vi "Begin.vi"(11 "Image Size":T1=enum."160x120") -> (0 "error out":errorcluster)   [LabVIEW 2012]
doc: "Called before other user functions, this VI is expected to open initial I/O refnums, load in file data, and do all program initialization. Notice that the <B>error out</B> terminal is simply used for data flow. Wiring it to other structures or subVIs ensures that this VI runs first."
uses:
  <vilib>/Rock Robotics/WPI/Camera/WPI_CameraImageSize.ctl
  <vilib>/Rock Robotics/SystemInterfaces/DIO/FPGA_DIOPWMChannel.ctl
  <vilib>/Rock Robotics/WPI/Camera/WPI_CameraWhite Balance Values.ctl
  <vilib>/Rock Robotics/WPI/Camera/WPI_CameraExposure Values.ctl
  <vilib>/Rock Robotics/WPI/Camera/WPI_CameraFrameRate.ctl
  <vilib>/Rock Robotics/WPI/DriverStation/WPI_DriverStationRobotMode2.ctl
  <vilib>/Rock Robotics/WPI/Joystick/WPI_JoystickDeviceEnum.ctl
  <vilib>/Rock Robotics/SystemInterfaces/Typedef/FPGA_TypedefSolenoidModule.ctl
  <vilib>/Rock Robotics/WPI/Solenoid/WPI_SolenoidChannel.ctl
  <vilib>/Rock Robotics/WPI/Encoder/WPI_EncoderType.ctl
  <vilib>/Rock Robotics/SystemInterfaces/DIO/FPGA_DIOChannel.ctl
  <vilib>/Rock Robotics/SystemInterfaces/Typedef/FPGA_TypedefDigitalModule.ctl
  <vilib>/Rock Robotics/WPI/SafetyOutput/WPI_SafetyOutputConfigMenu.ctl
  <vilib>/Rock Robotics/WPI/RobotDrive/WPI_RobotDriveOpen2MotorWithJaguar.vi
  F:/Team 1699 2013 robot code/Team 1699 2013 Robot Project V1a/Robot Global Data.vi
  <vilib>/Rock Robotics/WPI/Solenoid/WPI_SolenoidOpenSingle.vi
  <vilib>/Rock Robotics/WPI/Counter/WPI_CounterDigitalInputToDigitalSource.vi
  <vilib>/Rock Robotics/WPI/MotorControl/WPI_MotorControlOpen Talon.vi
  <vilib>/Utility/config.llb/Read Key (Double).vi
  <vilib>/Rock Robotics/SystemInterfaces/DIO/FPGA_DIORelayChannel.ctl
  <vilib>/Utility/config.llb/NI_LVConfig.lvlib
panel:
  out "found?":bool
  out "1699-preferences.ini":string[][](array[string])
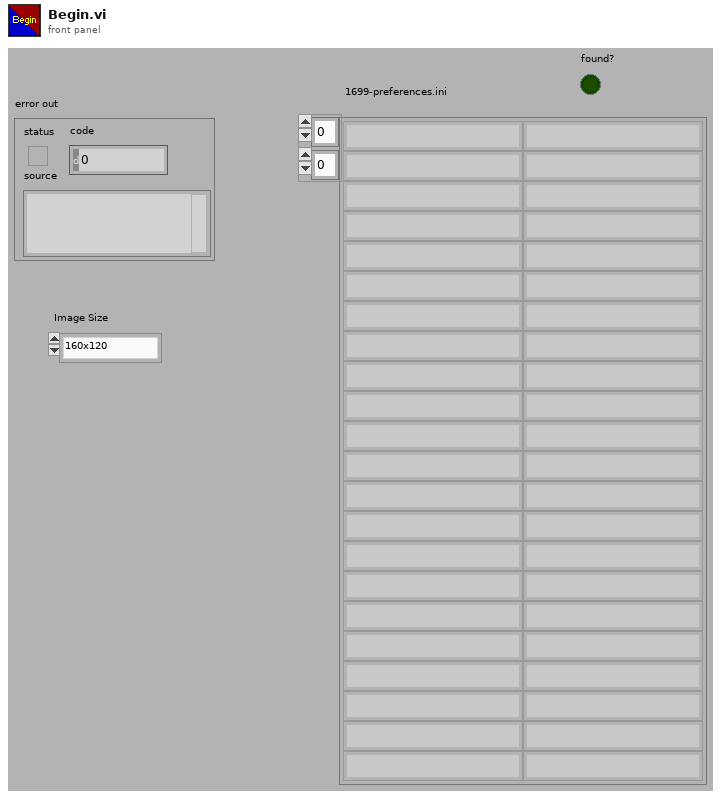
[diagram p1: front panel]
types:
  T1 = typedef "WPI_CameraImageSize.ctl" = enum16{"640x480", "320x240", "160x120"}
  T2 = typedef "WPI_SafetyOutputConfigMenu.ctl" = enum16{"Enable", "Disable"}
  T3 = typedef "FPGA_TypedefDigitalModule.ctl" = enum16{"Digital Module 1", "Digital Module 2"}
  T4 = typedef "FPGA_DIOPWMChannel.ctl" = enum8{"PWM 1", "PWM 2", "PWM 3", "PWM 4", "PWM 5", "PWM 6", "PWM 7", "PWM 8", "PWM 9", "PWM 10", "Invalid"}
  T5 = typedef "FPGA_DIOChannel.ctl" = enum8{"DIO 1", "DIO 2", "DIO 3", "DIO 4", "DIO 5", "DIO 6", "DIO 7", "DIO 8", "DIO 9", "DIO 10", "DIO 11", "DIO 12", "DIO 13", "DIO 14", "Invalid"}
  T6 = typedef "WPI_EncoderType.ctl" = enum16{"1x", "2x", "4x"}
  T7 = typedef "WPI_SolenoidChannel.ctl" = enum8{"Solenoid 1", "Solenoid 2", "Solenoid 3", "Solenoid 4", "Solenoid 5", "Solenoid 6", "Solenoid 7", "Solenoid 8", "Invalid"}
  T8 = typedef "FPGA_TypedefSolenoidModule.ctl" = enum16{"Solenoid Module 1", "Solenoid Module 2"}
  T9 = typedef "WPI_JoystickDeviceEnum.ctl" = enum16{"USB 1", "USB 2", "USB 3", "USB 4", "Kinect 1", "Kinect 2"}
  T10 = typedef "WPI_DriverStationRobotMode2.ctl" = enum16{"Autonomous Disabled", "Autonomous Enabled", "Teleop Disabled", "Teleop Enabled", "Timeout", "Finish", "Test Disabled", "Test Enabled"}
  T11 = typedef "WPI_CameraFrameRate.ctl" = u32
  T12 = typedef "WPI_CameraExposure Values.ctl" = enum16{"Auto", "Flicker-free 50 Hz", "Flicker-free 60 Hz", "Hold current"}
  T13 = typedef "WPI_CameraWhite Balance Values.ctl" = enum16{"Auto", "Fixed indoor", "Fixed outdoor 1", "Fixed outdoor 2", "Fixed fluorescent 1", "Fixed fluorescent 2", "Hold current"}
  T14 = typedef "WPI_DigitalInputDevRef.ctl" = cluster{"DevStatus":errorcluster, "DIO Channel":T5, "Digital Module":T3}
  T15 = typedef "FPGA_CounterEncoderSourceConvertionLVSourceType.ctl" = cluster{"DevStatus":errorcluster, "AnalogTriggerMode?":bool, "DigitalMode":cluster{"Digital Module":T3, "DIO Channel":T16}, "AnalogTriggerMode":cluster{"AnalogTriggerIndex":T17, "OutputType":T18}}
  T16 = typedef "FPGA_DIODigitalSourceChannel.ctl" = enum8{"DIO 1", "DIO 2", "DIO 3", "DIO 4", "DIO 5", "DIO 6", "DIO 7", "DIO 8", "DIO 9", "DIO 10", "DIO 11", "DIO 12", "DIO 13", "DIO 14", "Disabled"}
  T17 = typedef "FPGA_AnalogTriggerIndex.ctl" = enum8{"Trig 0", "Trig 1", "Trig 2", "Trig 3", "Trig 4", "Trig 5", "Trig 6", "Trig 7", "Invalid"}
  T18 = typedef "FPGA_AnalogTriggerOutType.ctl" = enum16{"InWindow", "TriggerState", "Rising", "Falling"}
  T19 = typedef "WPI_EncoderDevRef.ctl" = cluster{"DevStatus":errorcluster, "EncoderIndex":T20, "CounterIndex":T21, "DistancePerCount":dbl, "Decoding Type":T6}
  T20 = typedef "FPGA_EncoderIdx.ctl" = enum8{"Enc 0", "Enc 1", "Enc 2", "Enc 3", "Invalid"}
  T21 = typedef "FPGA_CounterCtrSystemIndex.ctl" = enum8{"Ctr 0", "Ctr 1", "Ctr 2", "Ctr 3", "Ctr 4", "Ctr 5", "Ctr 6", "Ctr 7", "Invalid"}
  T22 = cluster{"[0]":dbl, "[1]":dbl, "[2]":dbl, "[3]":dbl, "[4]":dbl, "[5]":dbl, "[6]":dbl, "[7]":dbl, "[8]":dbl, "[9]":dbl, "[10]":dbl, "[11]":dbl, "[12]":dbl, "[13]":dbl, "[14]":dbl, "[15]":dbl, "[16]":dbl, "[17]":dbl, "[18]":dbl, "[19]":dbl}
  T23 = typedef "FPGA_DIORelayChannel.ctl" = enum8{"Relay 1", "Relay 2", "Relay 3", "Relay 4", "Relay 5", "Relay 6", "Relay 7", "Relay 8", "Invalid"}
  T24 = typedef "WPI_CompressorDevRef.ctl" = cluster{"DevStatus":errorcluster, "DigitalInputDevRef":T14, "RelayDevRef":T25}
  T25 = typedef "WPI_RelayDevRef.ctl" = cluster{"DevStatus":errorcluster, "Relay Channel":T23, "Digital Module":T3, "Relay Direction":T26}
  T26 = typedef "WPI_RelayDirection.ctl" = enum16{"Both directions", "Forward only", "Reverse only"}
  T27 = typedef "WPI_MotorControlDeviceRef.ctl" = cluster{"DeviceStatus":errorcluster, "Type":enum16{"PWM", "CAN"}, "PWM":cluster{"Digital Module":T3, "PWM Channel":T4, "DeadBand":T28}, "CAN":cluster{"Device Number":u8, "Control Mode":T29, "Semaphore":T30, "Max Vout":dbl}, "Invert":bool, "TransformRef":T31, "InvTransformRef":T31}
  T28 = typedef "WPI_PWMDeadband.ctl" = cluster{"Name":string, "maxPositivePwm":i32, "minPositivePwm":i32, "centerPwm":i32, "maxNegativePwm":i32, "minNegativePwm":i32, "angularRange":u16}
  T29 = typedef "WPI_CANJaguar_ControlMode.ctl" = enum8{"Percent VBus", "Current", "Speed", "Position", "Voltage"}
  T30 = typedef "Semaphore RefNum" = refnum<k1>
  T31 = typedef "WPI_PWMTransform_ConPane.ctl" = refnum<vi>
  T32 = typedef "NI_LVConfig.lvlib/Config Data RefNum.ctl" = refnum<k1>
  T33 = typedef "WPI_JoystickDevRef.ctl" = cluster{"Device":T9}
  T34 = typedef "WPI_CameraDevRef.ctl" = cluster{"Camera Address":string, "CameraStatus":errorcluster, "Acquire Image Notifier":refnum<notifier>}
  T35 = typedef "WPI_RobotDriveDevRef.ctl" = cluster{"DevStatus":errorcluster, "Motors[]":T27[], "Square Inputs":bool, "Max Output":dbl, "Isochronous":bool}
  T36 = typedef "WPI_SolenoidDevRef.ctl" = cluster{"DevStatus":errorcluster, "Solenoid Module":T8, "Forward Solenoid Channel":T7, "Reverse Solenoid Channel":T7}
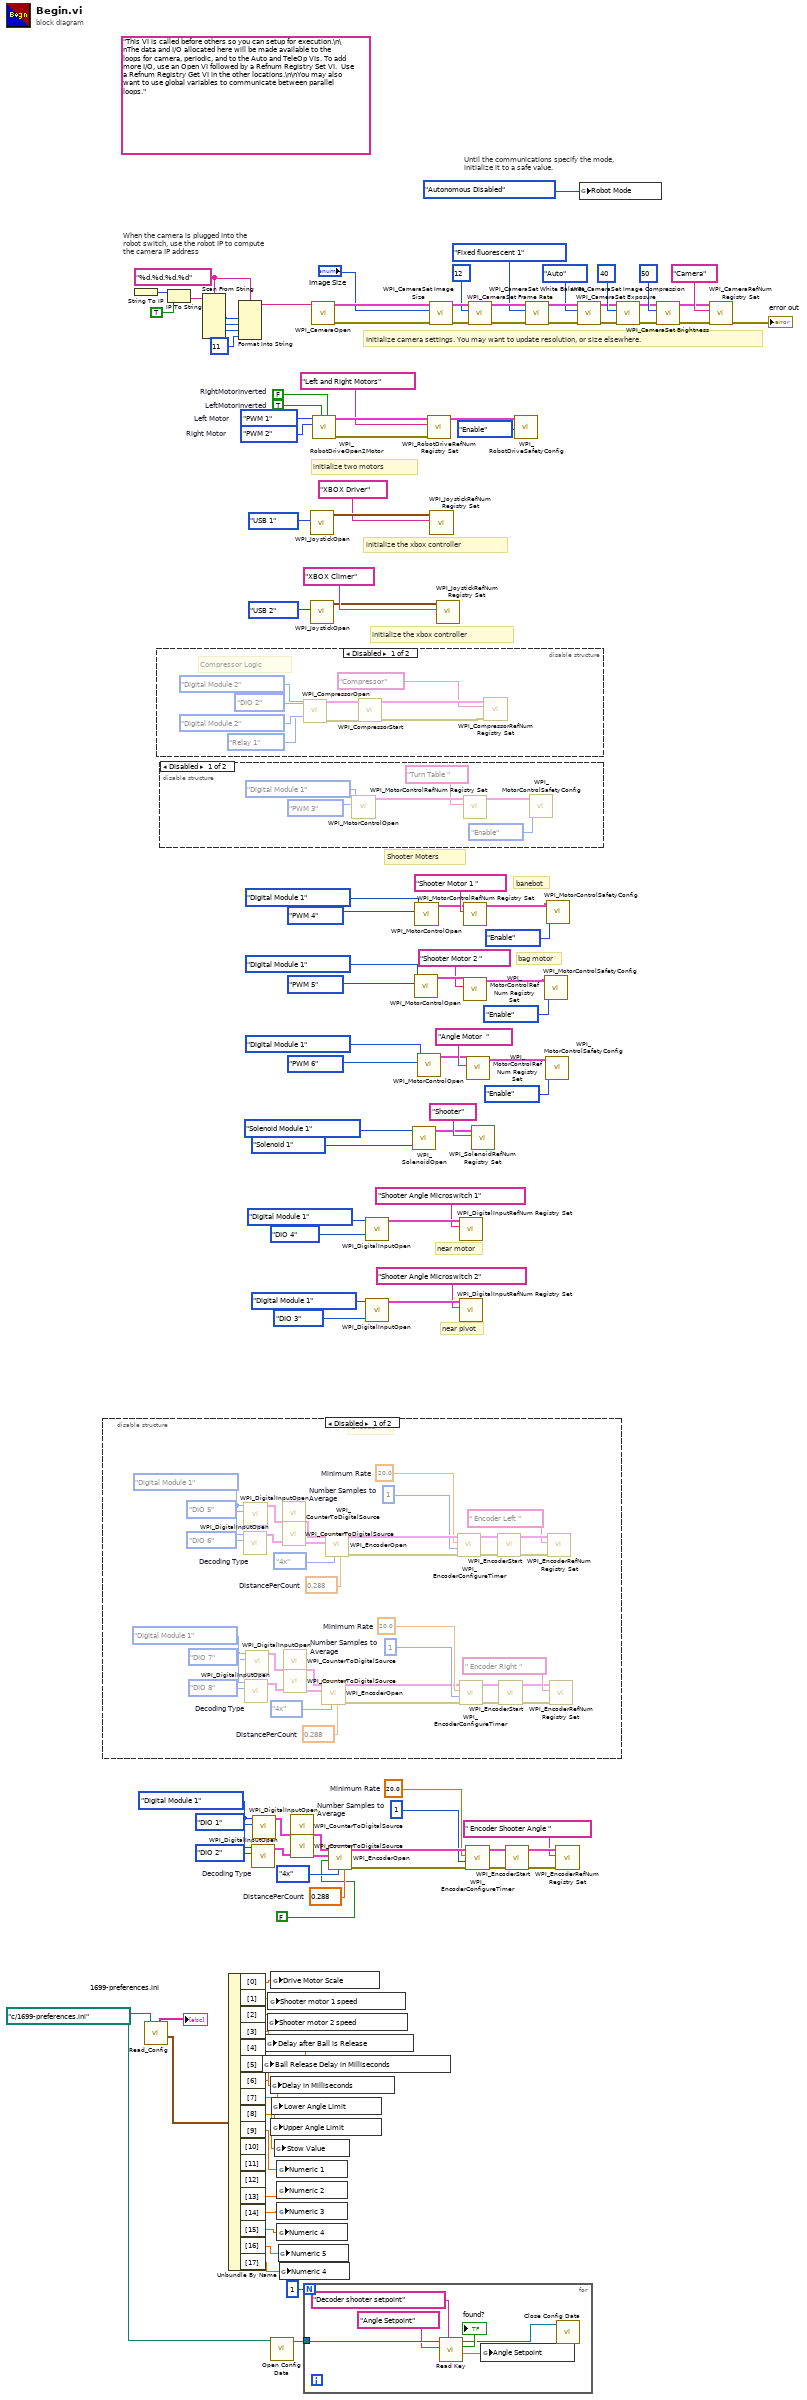
[diagram p0: block diagram]
diagram:
  w10 = path "c:/1699-preferences.ini" ("configuration file path")
  w48 = FPGA_TypedefDigitalModule."Digital Module 1" ("Digital Module (Module 1)")
  w55 = 0.288  # DistancePerCount
  w56 = WPI_EncoderType."4x"  # Decoding Type
  w57 = u8 1  # Number Samples to Average
  w58 = 20.0  # Minimum Rate
  w81 = "%d.%d.%d.%d" ("format string")
  (unwired) "This VI is called before others so you can setup for execution.\n\nThe data and I/O allocated here will be made available to the loops for camera, periodic, and to the Auto and TeleOp VIs. To add more I/O, use an Open VI followed by a Refnum Registry Set VI.  Use a Refnum Registry Get VI in the other locations.\n\nYou may also want to use global variables to communicate between parallel loops."
  w92 = FPGA_DIOPWMChannel."PWM 2"  # Right Motor
  w93 = FPGA_DIOPWMChannel."PWM 1"  # Left Motor
  w115 = TRUE  # LeftMotorInverted
  w116 = FALSE  # RightMotorInverted
  # "banebot"
  # "bag motor"
  # "Shooter Moters"
  # "initialize the xbox controller"
  # "near motor"
  # "near pivot"
  # "initialize the xbox controller"
  # "Until the communications specify the mode,\ninitialize it to a safe value."
  # "When the camera is plugged into the\nrobot switch, use the robot IP to compute\nthe camera IP address"
  # "initialize two motors"
  # "Initialize camera settings. You may want to update resolution, or size elsewhere."
  n1 = disable-structure shown="Disabled" {
    frame Disabled {
      w134 = FPGA_TypedefDigitalModule."Digital Module 1" ("Digital Module (Module 1)")
      w127 = 0.288  # DistancePerCount
      w126 = WPI_EncoderType."4x"  # Decoding Type
      w125 = u8 1  # Number Samples to Average
      w124 = 20.0  # Minimum Rate
      w135 = FPGA_TypedefDigitalModule."Digital Module 1" ("Digital Module (Module 1)")
      w142 = 0.288  # DistancePerCount
      w143 = WPI_EncoderType."4x"  # Decoding Type
      w144 = u8 1  # Number Samples to Average
      w145 = 20.0  # Minimum Rate
      # "Encoder"
      n2 = call <vilib>:"WPI_DigitalInputOpen.vi"("DIO Channel"=FPGA_DIOChannel."DIO 6", "Digital Module (Module 1)"=w135) -> ("DigitalInputDevRef"=w139:T14)  [unwired: 8 in, 1 out]
      n3 = call <vilib>:"WPI_DigitalInputOpen.vi"("DIO Channel"=FPGA_DIOChannel."DIO 5", "Digital Module (Module 1)"=w135) -> ("DigitalInputDevRef"=w138:T14)  [unwired: 8 in, 1 out]
      n4 = call <vilib>:"WPI_DigitalInputOpen.vi"("DIO Channel"=FPGA_DIOChannel."DIO 8", "Digital Module (Module 1)"=w134) -> ("DigitalInputDevRef"=w130:T14)  [unwired: 8 in, 1 out]
      n5 = call <vilib>:"WPI_DigitalInputOpen.vi"("DIO Channel"=FPGA_DIOChannel."DIO 7", "Digital Module (Module 1)"=w134) -> ("DigitalInputDevRef"=w131:T14)  [unwired: 8 in, 1 out]
      n6 = call-poly <vilib>:"WPI_CounterToDigitalSource.vi"("DigitalInputDevRef"=w138) -> ("Digital Source"=w140:T15)  [unwired: 6 in]
      n7 = call-poly <vilib>:"WPI_CounterToDigitalSource.vi"("DigitalInputDevRef"=w139) -> ("Digital Source"=w141:T15)  [unwired: 6 in]
      n8 = call-poly <vilib>:"WPI_CounterToDigitalSource.vi"("DigitalInputDevRef"=w131) -> ("Digital Source"=w129:T15)  [unwired: 6 in]
      n9 = call-poly <vilib>:"WPI_CounterToDigitalSource.vi"("DigitalInputDevRef"=w130) -> ("Digital Source"=w128:T15)  [unwired: 6 in]
      n10 = call <vilib>:"WPI_EncoderOpen.vi"("DistancePerCount"=w127, "Decoding Type"=w126, "BSource"=w128, "ASource"=w129) -> ("error out"=w123:errorcluster, "EncoderDevRef"=w117:T19)  [unwired: 6 in]
      n11 = call <vilib>:"WPI_EncoderOpen.vi"("DistancePerCount"=w142, "Decoding Type"=w143, "BSource"=w141, "ASource"=w140) -> ("error out"=w146:errorcluster, "EncoderDevRef"=w152:T19)  [unwired: 6 in]
      n12 = call <vilib>:"WPI_EncoderConfigureTimer.vi"("error in (no error)"=w146, "Number Samples to Average"=w144, "Minimum Rate"=w145, "EncoderDevRef"=w152) -> ("error out"=w147:errorcluster, "EncoderDevRef"=w151:T19)  [unwired: 6 in]
      n13 = call <vilib>:"WPI_EncoderConfigureTimer.vi"("error in (no error)"=w123, "Number Samples to Average"=w125, "Minimum Rate"=w124, "EncoderDevRef"=w117) -> ("error out"=w122:errorcluster, "EncoderDevRef"=w118:T19)  [unwired: 6 in]
      n14 = call <vilib>:"WPI_EncoderStart.vi"("error in (no error)"=w147, "EncoderDevRef"=w151) -> ("error out"=w148:errorcluster, "EncoderDevRef"=w150:T19)  [unwired: 8 in]
      n15 = call <vilib>:"WPI_EncoderStart.vi"("error in (no error)"=w122, "EncoderDevRef"=w118) -> ("error out"=w121:errorcluster, "EncoderDevRef"=w119:T19)  [unwired: 8 in]
      n16 = call <vilib>:"WPI_EncoderRefNum Registry Set.vi"("error in (no error)"=w148, "refnum name"=" Encoder Left ", "EncoderDevRef"=w150) -> ()  [unwired: 7 in, 2 out]
      n17 = call <vilib>:"WPI_EncoderRefNum Registry Set.vi"("error in (no error)"=w121, "refnum name"=" Encoder Right ", "EncoderDevRef"=w119) -> ()  [unwired: 7 in, 2 out]
    }
    frame Enabled {
    }
  }
  n18 = String To IP() -> (0:w88:u32)  [unwired: 1 in]
  n19 = call "Read_Config.vi"("configuration file path"=w10) -> ("PID Out"=w25:T22, "Array"=→"1699-preferences.ini":string[][])  [unwired: 2 in, 2 out]
  n20 = disable-structure shown="Disabled" {
    frame Disabled {
      # "Compressor Logic"
      n21 = call <vilib>:"WPI_CompressorOpen.vi"("Pressure Switch Digital Module (Module 1)"=FPGA_TypedefDigitalModule."Digital Module 2", "Pressure Switch DIO Channel"=FPGA_DIOChannel."DIO 2", "Relay Digital Module (Module 1)"=FPGA_TypedefDigitalModule."Digital Module 2", "Relay Channel"=FPGA_DIORelayChannel."Relay 1") -> ("CompressorDevRef"=w161:T24, "error out"=w160:errorcluster)  [unwired: 10 in]
      n22 = call <vilib>:"WPI_CompressorStart.vi"("error in (no error)"=w160, "CompressorDevRef"=w161) -> ("error out"=w159:errorcluster, "CompressorDevRef"=w158:T24)  [unwired: 8 in]
      n23 = call <vilib>:"WPI_CompressorRefNum Registry Set.vi"("error in (no error)"=w159, "refnum name"="Compressor", "CompressorDevRef"=w158) -> ()  [unwired: 7 in, 2 out]
    }
    frame Enabled {
    }
  }
  n24 = disable-structure shown="Disabled" {
    frame Disabled {
      n25 = call-poly <vilib>:"WPI_MotorControlOpen.vi"("PWM Channel"=FPGA_DIOPWMChannel."PWM 3", "Digital Module (Module 1)"=FPGA_TypedefDigitalModule."Digital Module 1") -> ("MotorControlDeviceRef"=w166:T27)  [unwired: 8 in, 1 out]
      n26 = call <vilib>:"WPI_MotorControlRefNum Registry Set.vi"("refnum name"="Turn Table ", "MotorControlDevRef"=w166) -> ("MotorControlDevRef"=w162:T27)  [unwired: 8 in, 1 out]
      n27 = call <vilib>:"WPI_MotorControlSafetyConfig.vi"("mode"=WPI_SafetyOutputConfigMenu."Enable", "MotorControlDevRef"=w162) -> ()  [unwired: 8 in, 2 out]
    }
    frame Enabled {
    }
  }
  n28 = IP To String(1:TRUE ("dot notation? (F)"), 2:w88) -> (0:w86:string)
  n29 = Scan From String(format string=w81, input string=w86) -> (output 1=w85:i32, output 2=w84:i32, output 3=w83:i32)  [unwired: 7 in, 3 out]
  n30 = Unbundle By Name(w25) -> ("[0]"=w24:dbl, "[1]"=w23:dbl, "[2]"=w22:dbl, "[3]"=w21:dbl, "[4]"=w20:dbl, "[5]"=w19:dbl, "[6]"=w18:dbl, "[7]"=w17:dbl, "[8]"=w16:dbl, "[9]"=w15:dbl, "[13]"=w14:dbl, "[14]"=w13:dbl, "[15]"=w12:dbl, "[16]"=w8:dbl, "[17]"=w7:dbl)  [unwired: 3 out]
  n31 = Format Into String(format string=w81, w85, w84, w83, 11 ("Compression")) -> (resulting string=w77:string)  [unwired: 2 in, 1 out]
  n32 = call <vilib>:"WPI_DigitalInputOpen.vi"("DIO Channel"=FPGA_DIOChannel."DIO 2", "Digital Module (Module 1)"=w48) -> ("DigitalInputDevRef"=w52:T14)  [unwired: 8 in, 1 out]
  n33 = call <vilib>:"WPI_DigitalInputOpen.vi"("DIO Channel"=FPGA_DIOChannel."DIO 1", "Digital Module (Module 1)"=w48) -> ("DigitalInputDevRef"=w51:T14)  [unwired: 8 in, 1 out]
  n34 = global write "Robot Global Data.vi" "Ball Release Delay in Milliseconds"(w20) -> ()
  n35 = global write "Robot Global Data.vi" "Delay after Ball is Release"(w21) -> ()
  n36 = global write "Robot Global Data.vi" "Shooter motor 2 speed"(w22) -> ()
  n37 = global write "Robot Global Data.vi" "Shooter motor 1 speed"(w23) -> ()
  n38 = global write "Robot Global Data.vi" "Delay in Milliseconds"(w19) -> ()
  n39 = call <vilib>:"Open Config Data.vi"("configuration file path"=w10) -> ("refnum"=w11:T32)  [unwired: 8 in, 2 out]
  n40 = global write "Robot Global Data.vi" "Drive Motor Scale"(w24) -> ()
  n41 = global write "Robot Global Data.vi" "Upper Angle Limit"(w17) -> ()
  n42 = global write "Robot Global Data.vi" "Lower Angle Limit"(w18) -> ()
  n43 = global write "Robot Global Data.vi" "Stow Value"(w16) -> ()
  n44 = global write "Robot Global Data.vi" "Numeric 1"(w15) -> ()
  n45 = global write "Robot Global Data.vi" "Numeric 2"(w14) -> ()
  n46 = global write "Robot Global Data.vi" "Numeric 3"(w13) -> ()
  n47 = global write "Robot Global Data.vi" "Numeric 4"(w12) -> ()
  n48 = global write "Robot Global Data.vi" "Numeric 5"(w8) -> ()
  n49 = global write "Robot Global Data.vi" "Numeric 4"(w7) -> ()
  n50 = call-poly <vilib>:"WPI_CounterToDigitalSource.vi"("DigitalInputDevRef"=w51) -> ("Digital Source"=w53:T15)  [unwired: 6 in]
  n51 = call-poly <vilib>:"WPI_CounterToDigitalSource.vi"("DigitalInputDevRef"=w52) -> ("Digital Source"=w54:T15)  [unwired: 6 in]
  n52 = for {
    N: 1 -> [_]
    tunnel: w11 -> [w173]
    n53 = call-poly <vilib>:"Read Key.vi"("section"="Decoder shooter setpoint", "key"="Angle Setpoint", "refnum"=w173) -> ("value"=w170:dbl, "found?"=→"found?":bool, "refnum out"=w168:T32)  [unwired: 5 in, 1 out]
    n54 = global write "Robot Global Data.vi" "Angle Setpoint"(w170) -> ()
    n55 = call <vilib>:"Close Config Data.vi"("refnum"=w168) -> ()  [unwired: 2 in, 9 out]
  }
  n56 = call <vilib>:"WPI_JoystickOpen.vi"("JoystickDevice"=WPI_JoystickDeviceEnum."USB 1") -> ("JoystickDevRef"=w72:T33)  [unwired: 10 out]
  n57 = call <vilib>:"WPI_JoystickOpen.vi"("JoystickDevice"=WPI_JoystickDeviceEnum."USB 2") -> ("JoystickDevRef"=w73:T33)  [unwired: 10 out]
  n58 = call <vilib>:"WPI_CameraOpen.vi"("Camera Address"=w77) -> ("error out"=w102:errorcluster, "CameraDevRef"=w103:T34)  [unwired: 1 in, 8 out]
  n59 = call-poly <vilib>:"WPI_RobotDriveOpen2Motor.vi"("Right Motor Inverted"=w116, "Left Motor Inverted"=w115, "Right Motor"=w92, "Left Motor"=w93) -> ("error out"=w111:errorcluster, "RobotDriveDevRef"=w113:T35)  [unwired: 1 in, 5 out]
  n60 = call <vilib>:"WPI_EncoderOpen.vi"("DistancePerCount"=w55, "Decoding Type"=w56, "Invert Direction (False)"=FALSE, "BSource"=w54, "ASource"=w53) -> ("error out"=w59:errorcluster, "EncoderDevRef"=w65:T19)  [unwired: 5 in]
  n61 = call <vilib>:"WPI_DigitalInputOpen.vi"("DIO Channel"=FPGA_DIOChannel."DIO 4", "Digital Module (Module 1)"=FPGA_TypedefDigitalModule."Digital Module 1") -> ("DigitalInputDevRef"=w42:T14)  [unwired: 1 in, 8 out]
  n62 = call <vilib>:"WPI_DigitalInputOpen.vi"("DIO Channel"=FPGA_DIOChannel."DIO 3", "Digital Module (Module 1)"=FPGA_TypedefDigitalModule."Digital Module 1") -> ("DigitalInputDevRef"=w43:T14)  [unwired: 1 in, 8 out]
  n63 = call-poly <vilib>:"WPI_SolenoidOpen.vi"("Solenoid Channel"=WPI_SolenoidChannel."Solenoid 1", "Solenoid Module (Module 1)"=FPGA_TypedefSolenoidModule."Solenoid Module 1") -> ("SolenoidDevRef"=w66:T36)  [unwired: 8 in, 1 out]
  n64 = call-poly <vilib>:"WPI_MotorControlOpen.vi"("PWM Channel"=FPGA_DIOPWMChannel."PWM 5", "Digital Module (Module 1)"=FPGA_TypedefDigitalModule."Digital Module 1") -> ("MotorControlDeviceRef"=w37:T27)  [unwired: 8 in, 1 out]
  n65 = call-poly <vilib>:"WPI_MotorControlOpen.vi"("PWM Channel"=FPGA_DIOPWMChannel."PWM 4", "Digital Module (Module 1)"=FPGA_TypedefDigitalModule."Digital Module 1") -> ("MotorControlDeviceRef"=w34:T27)  [unwired: 8 in, 1 out]
  n66 = call-poly <vilib>:"WPI_MotorControlOpen.vi"("PWM Channel"=FPGA_DIOPWMChannel."PWM 6", "Digital Module (Module 1)"=FPGA_TypedefDigitalModule."Digital Module 1") -> ("MotorControlDeviceRef"=w29:T27)  [unwired: 8 in, 1 out]
  n67 = call <vilib>:"WPI_RobotDriveRefNum Registry Set.vi"("error in (no error)"=w111, "refnum name"="Left and Right Motors", "RobotDriveDevRef"=w113) -> ("RobotDriveDevRef"=w80:T35)  [unwired: 8 out]
  n68 = call <vilib>:"WPI_CameraSet Image Size.vi"("error in (no error)"=w102, "Image Size"="Image Size", "CameraDevRef"=w103) -> ("error out"=w101:errorcluster, "CameraDevRef Out"=w104:T34)  [unwired: 7 out]
  n69 = call <vilib>:"WPI_JoystickRefNum Registry Set.vi"("refnum name"="XBOX Driver", "JoystickDevRef"=w72) -> ()  [unwired: 1 in, 9 out]
  n70 = call <vilib>:"WPI_JoystickRefNum Registry Set.vi"("refnum name"="XBOX Climer", "JoystickDevRef"=w73) -> ()  [unwired: 1 in, 9 out]
  n71 = call <vilib>:"WPI_DigitalInputRefNum Registry Set.vi"("refnum name"="Shooter Angle Microswitch 1", "DigitalInputDevRef"=w42) -> ()  [unwired: 8 in, 2 out]
  n72 = call <vilib>:"WPI_DigitalInputRefNum Registry Set.vi"("refnum name"="Shooter Angle Microswitch 2", "DigitalInputDevRef"=w43) -> ()  [unwired: 8 in, 2 out]
  n73 = call <vilib>:"WPI_MotorControlRefNum Registry Set.vi"("refnum name"="Shooter Motor 1 ", "MotorControlDevRef"=w34) -> ("MotorControlDevRef"=w1:T27)  [unwired: 8 in, 1 out]
  n74 = call <vilib>:"WPI_MotorControlRefNum Registry Set.vi"("refnum name"="Shooter Motor 2 ", "MotorControlDevRef"=w37) -> ("MotorControlDevRef"=w2:T27)  [unwired: 8 in, 1 out]
  n75 = call <vilib>:"WPI_EncoderConfigureTimer.vi"("error in (no error)"=w59, "Number Samples to Average"=w57, "Minimum Rate"=w58, "EncoderDevRef"=w65) -> ("error out"=w60:errorcluster, "EncoderDevRef"=w64:T19)  [unwired: 6 in]
  n76 = call <vilib>:"WPI_MotorControlRefNum Registry Set.vi"("refnum name"="Angle Motor  ", "MotorControlDevRef"=w29) -> ("MotorControlDevRef"=w3:T27)  [unwired: 8 in, 1 out]
  n77 = call <vilib>:"WPI_CameraSet Frame Rate.vi"("error in (no error)"=w101, "Frame Rate (fps)"=T11 12, "CameraDevRef"=w104) -> ("error out"=w100:errorcluster, "CameraDevRef Out"=w106:T34)  [unwired: 7 out]
  n78 = call <vilib>:"WPI_SolenoidRefNum Registry Set.vi"("refnum name"="Shooter", "SolenoidDevRef"=w66) -> ()  [unwired: 8 in, 2 out]
  n79 = call <vilib>:"WPI_EncoderStart.vi"("error in (no error)"=w60, "EncoderDevRef"=w64) -> ("error out"=w61:errorcluster, "EncoderDevRef"=w63:T19)  [unwired: 8 in]
  n80 = call <vilib>:"WPI_RobotDriveSafetyConfig.vi"("mode"=WPI_SafetyOutputConfigMenu."Enable", "RobotDriveDevRef"=w80) -> ()  [unwired: 8 in, 2 out]
  n81 = call <vilib>:"WPI_CameraSet White Balance.vi"("error in (no error)"=w100, "White Balance"=WPI_CameraWhite_Balance_Values."Fixed fluorescent 1", "CameraDevRef"=w106) -> ("error out"=w99:errorcluster, "CameraDevRef Out"=w105:T34)  [unwired: 7 out]
  n82 = call <vilib>:"WPI_MotorControlSafetyConfig.vi"("mode"=WPI_SafetyOutputConfigMenu."Enable", "MotorControlDevRef"=w2) -> ()  [unwired: 8 in, 2 out]
  n83 = call <vilib>:"WPI_MotorControlSafetyConfig.vi"("mode"=WPI_SafetyOutputConfigMenu."Enable", "MotorControlDevRef"=w3) -> ()  [unwired: 8 in, 2 out]
  n84 = call <vilib>:"WPI_MotorControlSafetyConfig.vi"("mode"=WPI_SafetyOutputConfigMenu."Enable", "MotorControlDevRef"=w1) -> ()  [unwired: 8 in, 2 out]
  n85 = call <vilib>:"WPI_EncoderRefNum Registry Set.vi"("error in (no error)"=w61, "refnum name"=" Encoder Shooter Angle ", "EncoderDevRef"=w63) -> ()  [unwired: 7 in, 2 out]
  n86 = call <vilib>:"WPI_CameraSet Exposure.vi"("error in (no error)"=w99, "Exposure"=WPI_CameraExposure_Values."Auto", "CameraDevRef"=w105) -> ("error out"=w98:errorcluster, "CameraDevRef Out"=w108:T34)  [unwired: 7 out]
  n87 = global write "Robot Global Data.vi" "Robot Mode"(WPI_DriverStationRobotMode2."Autonomous Disabled" ("Robot Mode")) -> ()
  n88 = call <vilib>:"WPI_CameraSet Image Compression.vi"("error in (no error)"=w98, "Compression"=40, "CameraDevRef"=w108) -> ("error out"=w97:errorcluster, "CameraDevRef Out"=w107:T34)  [unwired: 7 out]
  n89 = call <vilib>:"WPI_CameraSet Brightness.vi"("error in (no error)"=w97, "Brightness"=50, "CameraDevRef"=w107) -> ("error out"=w95:errorcluster, "CameraDevRef Out"=w96:T34)  [unwired: 7 out]
  n90 = call <vilib>:"WPI_CameraRefNum Registry Set.vi"("error in (no error)"=w95, "refnum name"="Camera", "CameraDevRef"=w96) -> ("error out"=→"error out":errorcluster)  [unwired: 8 out]
